vi "Handle.vi"(7 "Queue Actor in":refnum<class "Queue Actor.lvclass">, 11 "Teardown Queue State in":refnum<class "Teardown Queue State.lvclass">) -> (2 "Destroy?":bool, 5 "Queue Actor out":refnum<class "Queue Actor.lvclass">)   [LabVIEW 2021, in "jettl.lvlib" / "Teardown Queue State.lvclass"]
uses:
  Teardown Queue State.lvclass
  Queue Actor/Queue Actor.lvclass
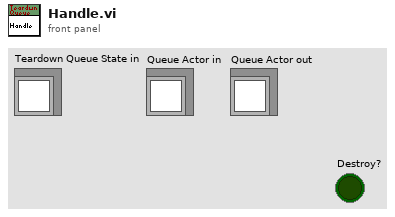
[diagram p1: front panel]
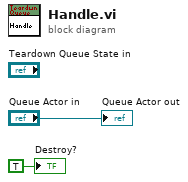
[diagram p0: block diagram]
diagram:
  "Destroy?" <- TRUE ("Destroy?")
  "Queue Actor out" <- "Queue Actor in"
